vi "Activate Devices.vi"(6 "stop":refnum<notifier>, 8 "error in":errorcluster, 11 "Activation in":refnum<class "Activation.lvclass">) -> (0 "error out":errorcluster, 2 "Failed Devices":T1[](array[typedef]), 3 "Activation out":refnum<class "Activation.lvclass">, 4 "Activation Failed?":bool)   [LabVIEW 2018, in "Startup Optimization Actor.lvlib" / "Startup Optimization.lvclass"]
uses:
  Startup Optimization.lvclass
  Activation Actor/Activation/Activation.lvclass
  C:/Users/Administrator/Desktop/LabVIEW EMS/Optimization/Startup Optimization Actor/Startup Optimization/Startup Optimization.lvclass
  C:/Users/Administrator/Desktop/LabVIEW EMS/EMS Generic Actor/EMS Generic/EMS Generic.lvclass
  C:/Users/Administrator/Desktop/LabVIEW EMS/Device Communication and Control Abstract Actor/Device Communication and Control Abstract/Device Communication and Control Abstract.lvclass
  <vilib>/ORNL/CSEISMIC DDS/CSEISMIC DDS Base/Data Types/Controls/DeviceID.ctl
  Startup Optimization.lvclass/Startup Optimization.ctl
  EMS Generic Actor/EMS Generic/EMS Generic.lvclass/EMS Generic.ctl
  <vilib>/ORNL/CSEISMIC DDS/CSEISMIC DDS Base/Data Types/DER_Control.ctl
  <vilib>/ActorFramework/Actor/Actor.lvclass/Actor.ctl
  Device Communication and Control Abstract Actor/Device Communication and Control Abstract/Device Communication and Control Abstract.lvclass/Device Communication and Control Abstract.ctl
  Device Communication and Control Abstract Actor/Device Communication and Control Abstract Messages/Set DER Control Msg/Set DER Control Msg.lvclass/Set DER Control Msg.ctl
  <vilib>/ActorFramework/Message Enqueuer/Message Enqueuer.lvclass/Message Enqueuer.ctl
  Device Communication and Control Abstract Actor/Device Communication and Control Abstract Messages/Set DER Control Msg/Send Set DER Control.vi
  <vilib>/ActorFramework/Actor/Read Caller Enqueuer.vi
  <vilib>/ActorFramework/Message Enqueuer/Enqueue.vi
  Device Communication and Control Abstract Actor/Device Communication and Control Abstract/Device Communication and Control Abstract.lvclass
  C:/Program Files (x86)/National Instruments/LabVIEW 2018/vi.lib/ActorFramework/Actor/Actor.lvclass
  Device Communication and Control Abstract Actor/Device Communication and Control Abstract Messages/Set DER Control Msg/Set DER Control Msg.lvclass
  C:/Program Files (x86)/National Instruments/LabVIEW 2018/vi.lib/ActorFramework/Message/Message.lvclass
  <vilib>/ActorFramework/Message Priority Queue/Priority Enqueue.vi
  <vilib>/ORNL/CSEISMIC DDS/CSEISMIC DDS Base/CSEISMIC DDS.lvclass
  EMS Generic Actor/EMS Generic/EMS Generic.lvclass
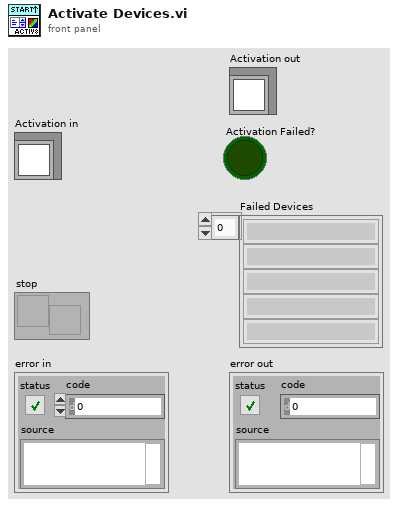
[diagram p1: front panel]
types:
  T1 = typedef "CSEISMIC DDS.lvlib/CSEISMIC DDS.lvclass/DeviceID.ctl" = string
  T2 = typedef "EMS Generic Actor.lvlib/EMS Generic.lvclass/Global Configuration.ctl" = cluster{"Microgrid ID":u8, "VF Device ID":T1, "Ongrid VF Priority":T1[], "Offgrid VF Priority":T1[], "AutoSwap Offgrid VF":u32, "AutoSwap Offgrid VF Delay (sec)":dbl, "AutoSwap Resynch VF":u32, "PCC Device ID":T1, "Device ID Array":T1[], "Nominal Voltage":dbl, "Nominal Frequency":dbl, "Resynch Timeout (sec)":dbl, "Island VF Activate Timeout (sec)":dbl, "Island PCC Target Power (kW)":dbl, "Island PCC Target Power Timeout (sec)":dbl, "Island Grid Settle Time (sec)":dbl, "Island PCC Failure Timeout (sec)":dbl, "Activation Devices Present Timeout (sec)":dbl, "Activation Devices Activated Timeout (sec)":dbl, "Blackstart VF GenMode Wait (sec)":dbl, "Blackstart VF DERCtrl Wait (sec)":dbl, "Blackstart Success Wait (sec)":dbl, "OnGrid Optimization Delay (sec)":dbl, "OffGrid Optimization Delay (sec)":dbl, "Resynch Frequency (Hz)":dbl, "Optimization Path":string}
  T3 = typedef "CSEISMIC DDS.lvlib/CSEISMIC DDS.lvclass/DER_Control.ctl" = cluster{"DeviceID":T1, "Activate":bool, "Deactivate":bool}
  T4 = typedef "CSEISMIC DDS.lvlib/CSEISMIC DDS.lvclass/IED_Status.ctl" = cluster{"DeviceID":T1, "Timestamp":T5, "MicrogridID":u8, "Active":bool, "Inactive":bool, "Error":i32, "Fault":bool, "ErrorString":string}
  T5 = typedef "CSEISMIC DDS.lvlib/CSEISMIC DDS.lvclass/Timestamp.ctl" = cluster{"Seconds":u64, "Remainder":u64}
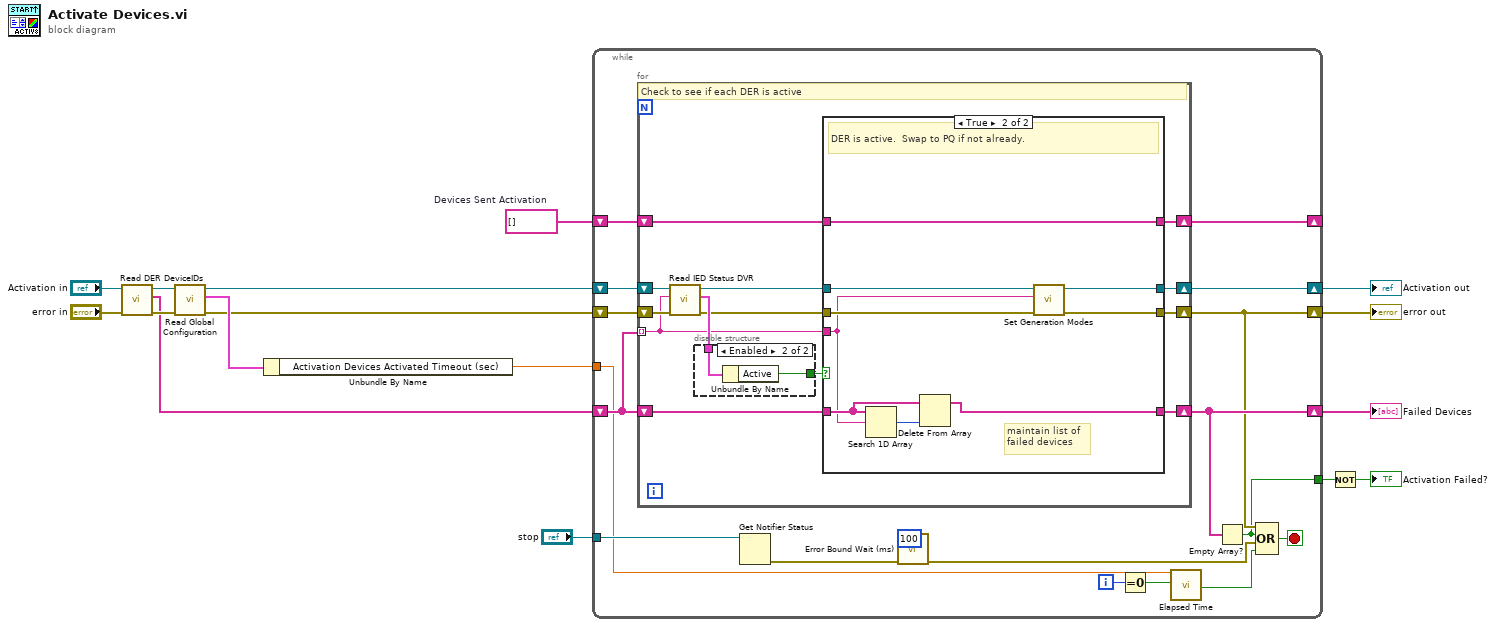
[diagram p0: block diagram]
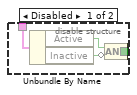
[diagram p2: hidden frame]
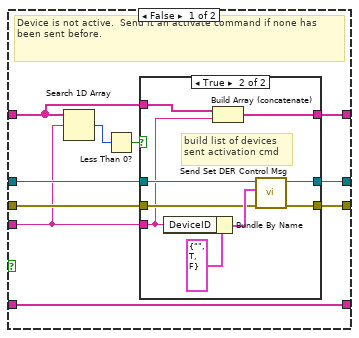
[diagram p3: hidden frame]
diagram:
  w8 = T1[] []  # Devices Sent Activation
  n1 = call "Read DER DeviceIDs.vi"("error in"="error in", "Startup Optimization in"="Activation in") -> ("error out"=w4:errorcluster, "DERs"=w1:T1[], "Startup Optimization out"=w6:refnum<class "Activation.lvclass">)  [unwired: 7 in]
  n2 = call "Read Global Configuration.vi"("error in"=w4, "EMS Generic in"=w6) -> ("error out"=w3:errorcluster, "Global Configuration"=w13:T2, "dup EMS Generic out"=w2:refnum<class "Activation.lvclass">)  [unwired: 7 in]
  n3 = Unbundle By Name(w13) -> ("Activation Devices Activated Timeout (sec)"=w12:dbl)
  n4 = while {
    shift-right: [w17] -> w15
    shift-left: w2 -> [w33]
    shift-right: [w28] -> w14
    shift-left: w3 -> [w34]
    shift-right: [w31] -> w9
    shift-left: w1 -> [w32]
    tunnel: "stop" -> [w30]
    tunnel: w12 -> [w21]
    tunnel: [w20] -> w11
    shift-right: [w18] -> _
    shift-left: w8 -> [w19]
    i -> [w23]
    stop <- w25 stop-if-true
    n5 = for {
      tunnel: w32 -> [w38] mode=indexing
      shift-right: [w46] -> w28
      shift-left: w34 -> [w42]
      shift-right: [w47] -> w17
      shift-left: w33 -> [w40]
      shift-right: [w44] -> w31
      shift-left: w32 -> [w45]
      shift-right: [w35] -> w18
      shift-left: w19 -> [w36]
      # "Check to see if each DER is active"
      n6 = call "Read IED Status DVR.vi"("error in"=w42, "DeviceID"=w38, "EMS Generic in"=w40) -> ("error out"=w41:errorcluster, "IED_Status"=w43:T4, "EMS Generic out"=w39:refnum<class "Activation.lvclass">)  [unwired: 5 in, 1 out]
      n7 = disable-structure shown="Enabled" {
        disable-tunnel: w43 -> [w51 w53]
        disable-tunnel: [w48 w52] -> w37
        frame Disabled {
          n8 = Unbundle By Name(w51) -> ("Active"=w50:bool, "Inactive"=w49:bool)
          n9 = Compound Arithmetic op=AND(w50, invert w49) -> (w48:bool)
        }
        frame Enabled {
          n10 = Unbundle By Name(w53) -> ("Active"=w52:bool)
        }
      }
      n11 = case shown="True" w37 {
        tunnel: w38 -> [w58 w76]
        tunnel: w41 -> [w62 w78]
        tunnel: w39 -> [w60 w79]
        tunnel: [w59 w84] -> w47
        tunnel: [w61 w83] -> w46
        tunnel: w45 -> [w63 w81]
        tunnel: [w63 w80] -> w44
        tunnel: w36 -> [w55 w77]
        tunnel: [w54 w77] -> w35
        frame False {
          # "Device is not active.  Send it an activate command if none has been sent before."
          n12 = Search 1D Array(1D array=w55, element=w58) -> (index of element=w57:i32)  [unwired: 1 in]
          n13 = Less Than 0?(x=w57) -> (x < 0?=w56:bool)
          n14 = case shown="True" w56 {
            tunnel: w62 -> [w64 w73]
            tunnel: [w64 w72] -> w61
            tunnel: w60 -> [w65 w71]
            tunnel: [w65 w70] -> w59
            tunnel: w58 -> [_ w68]
            tunnel: w55 -> [w66 w69]
            tunnel: [w66 w67] -> w54
            frame False {
              # "already sent activate cmd"
            }
            frame True {
              # "build list of devices sent activation cmd"
              n15 = Bundle By Name(cluster=T3 {"DeviceID"="", "Activate"=TRUE, "Deactivate"=FALSE} ("DER_Control"), "DeviceID"=w68) -> (w75:T3)
              n16 = Build Array (concatenate)(w69, w68) -> (w67:T1[])
              n17 = call "Send Set DER Control Msg.vi"("error in"=w73, "DER_Control"=w75, "SCADA Sub Abstract in"=w71) -> ("error out"=w72:errorcluster, "dup SCADA Sub Abstract"=w70:refnum<class "Activation.lvclass">)  [unwired: 7 in]
            }
          }
        }
        frame True {
          # "maintain list of failed devices"
          # "DER is active.  Swap to PQ if not already."
          n18 = Search 1D Array(1D array=w81, element=w76) -> (index of element=w82:i32)  [unwired: 1 in]
          n19 = Delete From Array(array=w81, index=w82) -> (array with subset deleted=w80:T1[])  [unwired: 1 in, 1 out]
          n20 = call "Set Generation Modes.vi"("error in"=w78, "DeviceID"=w76, "Activation in"=w79) -> ("error out"=w83:errorcluster, "Activation out"=w84:refnum<class "Activation.lvclass">)  [unwired: 7 in]
        }
      }
    }
    n21 = Get Notifier Status(notifier=w30) -> (error out=w29:errorcluster)  [unwired: 1 in, 4 out]
    n22 = call "Error Bound Wait (ms).vi"("milliseconds to wait (100)"=u32 100 ("milliseconds to wait"), "error in"=w29) -> ("error out"=w27:errorcluster)  [unwired: 9 in]
    n23 = Equal To 0?(x=w23) -> (x = 0?=w24:bool)
    n24 = call "Elapsed Time"("Time Target (s)"=w21, "Reset"=w24) -> ("Time has Elapsed"=w22:bool)  [unwired: 10 in, 7 out]
    n25 = Empty Array?(array=w31) -> (empty?=w20:bool)
    n26 = Compound Arithmetic op=OR(w28, w20, w27, w22) -> (w25:bool)
  }
  "Activation out" <- w15
  "error out" <- w14
  "Failed Devices" <- w9
  n27 = Not(x=w11) -> (.not. x?=→"Activation Failed?":bool)
